vi "BoolCmd_Send_BoolEdge.vi"(9 "Value":bool, 11 "Command Name":string) -> (0 "error out":errorcluster)   [LabVIEW 2019, in "Trajectory_Library.lvlib"]
uses:
  Trajectory_Library.lvlib
  BoolCmd_ObtainQueue.vi
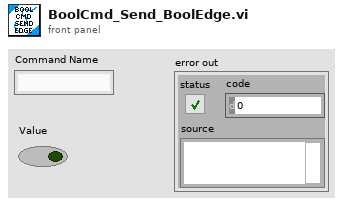
[diagram p1: front panel]
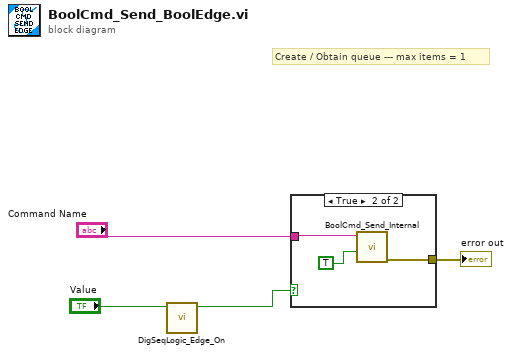
[diagram p0: block diagram]
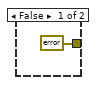
[diagram p2: hidden frame]
diagram:
  # "Create / Obtain queue --- max items = 1"
  n1 = call "DigSeqLogic_Edge_On.vi"("Input"="Value") -> ("On Edge"=w3:bool)  [unwired: 10 in]
  n2 = case shown="True" w3 {
    tunnel: "Command Name" -> [_ w8]
    tunnel: [errorcluster {"status"=FALSE, "code"=0, "source"=""} ("error out") w6] -> w1
    frame False {
    }
    frame True {
      n3 = call "BoolCmd_Send_Internal.vi"("Value"=TRUE, "Command Name"=w8) -> ("error out"=w6:errorcluster)  [unwired: 9 in]
    }
  }
  "error out" <- w1
